vi "CompileMaster.vi"(0 "Type":enum16{"Meta", "Aux", "Main"}(ring), 2 "Stepnum":i32, 3 "Compiler Settings":T1={"Python Path"=path "", "Main File"="scriptmain.py", "Meta File"="scriptmeta.txt", "Aux File"="scriptaux.py", "Pre File"="metascript.txt"}) -> (4 "CompileSuccess?":bool=TRUE, 5 "Params":T3, 6 "PulseList":T2[](array[typedef]), 7 "RF Array":variant[](array[variant]), 8 "standard output":string, 9 "Standard Error Out":string)   [LabVIEW 2019]
uses:
  Params.ctl
  SinglePulse.ctl
  PulseCompiler/CompilerSettings.ctl
  Log/GlobalPyConsole.vi
  Global.lvlib
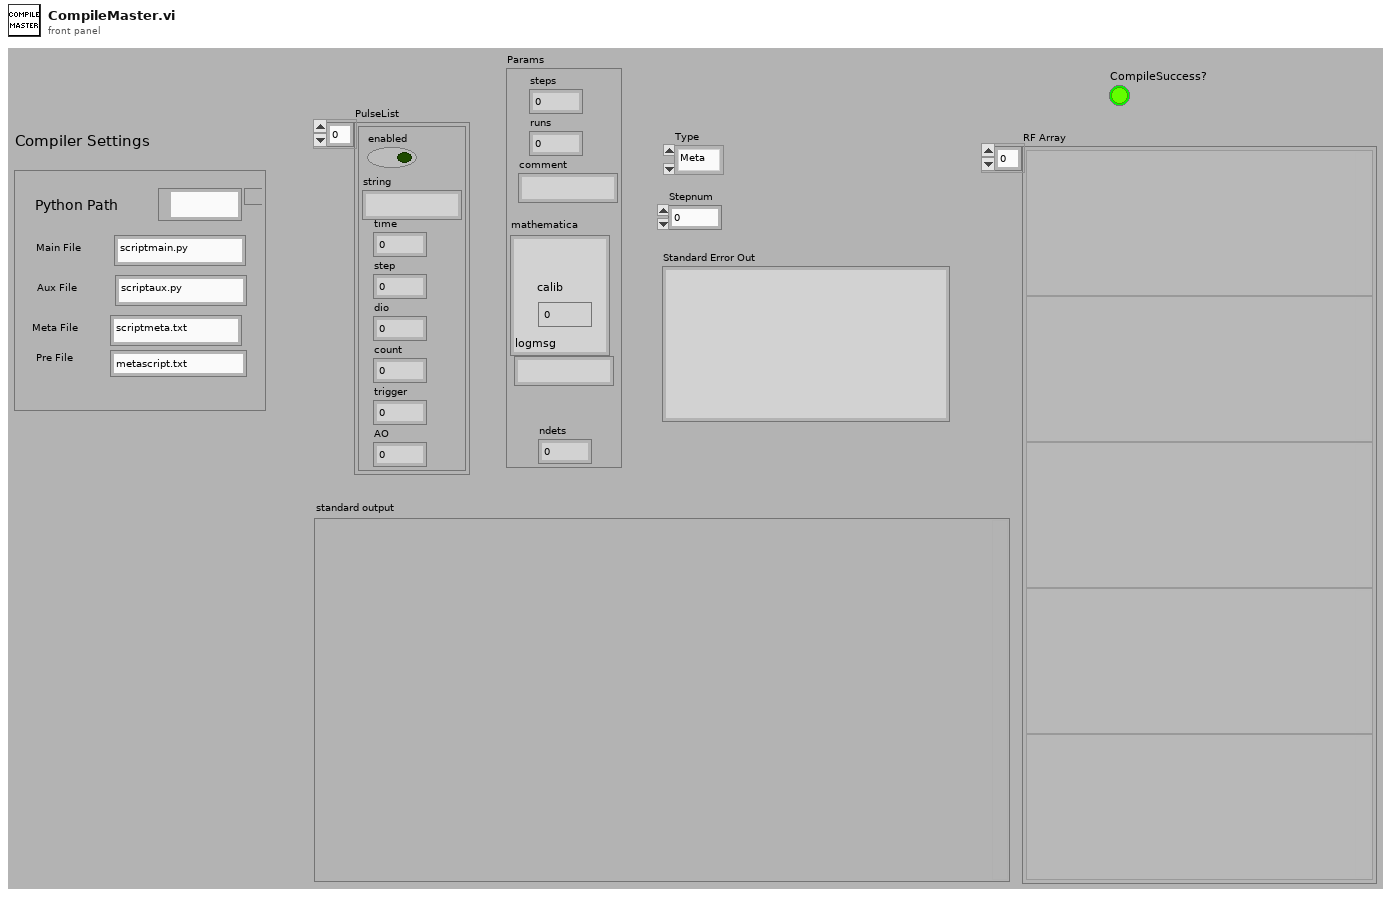
[diagram p1: front panel]
types:
  T1 = typedef "CompilerSettings.ctl" = cluster{"Python Path":path, "Main File":string, "Meta File":string, "Aux File":string, "Pre File":string}
  T2 = typedef "SinglePulse.ctl" = cluster{"enabled":bool, "string":string, "time":dbl, "step":dbl, "dio":dbl, "count":dbl, "trigger":dbl, "AO":dbl}
  T3 = typedef "Params.ctl" = cluster{"steps":i16, "runs":i16, "comment":string, "mathematica":string, "calib":i8, "logmsg":string, "ndets":i16}
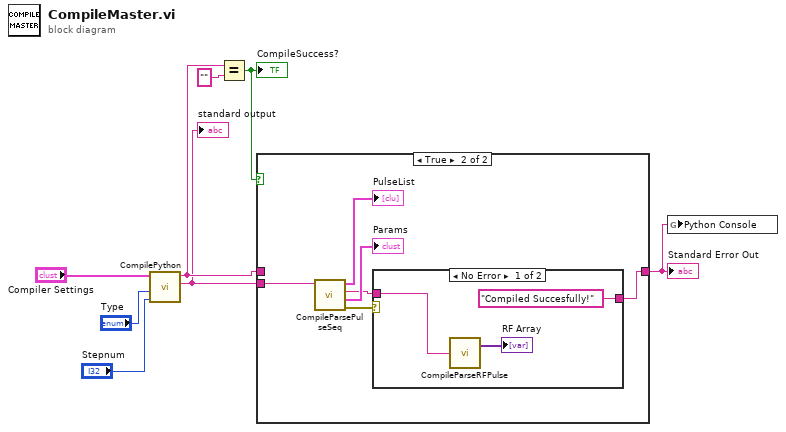
[diagram p0: block diagram]
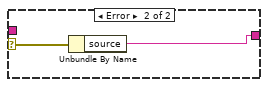
[diagram p3: hidden frame]
diagram:
  n1 = call "CompilePython.vi"("Stepnum"="Stepnum", "Enum"="Type", "Compiler Settings"="Compiler Settings") -> ("standard output"=w3:string, "standard error"=w5:string)  [unwired: 7 in]
  "standard output" <- w3
  n2 = Equal?(x=w5, y="") -> (x = y?=w4:bool)
  "CompileSuccess?" <- w4
  n3 = case shown="True" w4 {
    tunnel: w5 -> [w9 _]
    tunnel: w3 -> [_ w14]
    tunnel: [w9 w10] -> w1
    frame False {
    }
    frame True {
      n4 = call "CompileParsePulseSeq.vi"("PulseSeqIn"=w14) -> ("error out"=w11:errorcluster, "Params"=→"Params":T3, "RFPulseList"=w12:string, "PulseList"=→"PulseList":T2[])  [unwired: 7 in]
      n5 = case shown="No Error" w11 {
        selector: w11 -> [_ w20]
        tunnel: w12 -> [w17 _]
        tunnel: ["Compiled Succesfully!" ("standard error") w19] -> w10
        frame No Error {
          n6 = call "CompileParseRFPulse.vi"("String"=w17) -> ("Array"=→"RF Array":variant[])  [unwired: 1 in]
        }
        frame Error {
          n7 = Unbundle By Name(w20) -> ("source"=w19:string)
        }
      }
    }
  }
  "Standard Error Out" <- w1
  n8 = global write "GlobalPyConsole.vi" "Python Console"(w1) -> ()
